vi "GDSLvCLass_ReadClassPropertiesFromFile.vi"(0 "LvClassPathIn":path, 5 "error in (no error)":errorcluster) -> (14 "LvClassPathOut":path, 15 "ClassSettings":T1, 16 "DataFlowClass":bool, 19 "error out":errorcluster)   [LabVIEW 2020]
uses:
  GDSLvCLass_ClassSettingsType.ctl
  GDSLvClass_PlugIn.ctl
  GDSLvClass_PlugInTypes.ctl
  GDSLvClass_ClassTypeSettingNames.ctl
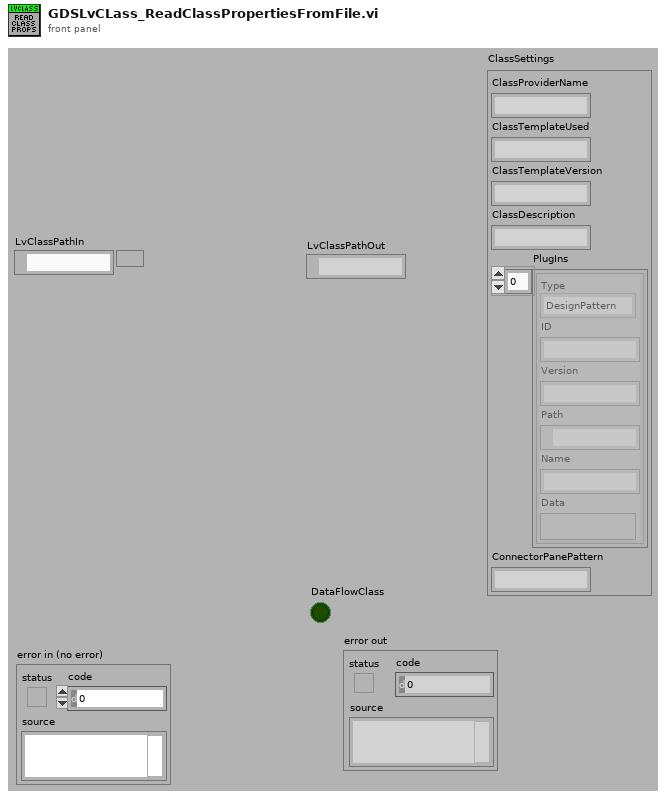
[diagram p1: front panel]
types:
  T1 = typedef "GDSLvCLass_ClassSettingsType.ctl" = cluster{"ClassProviderName":string, "ClassTemplateUsed":string, "ClassTemplateVersion":string, "ClassDescription":string, "PlugIns":T2[], "ConnectorPanePattern":string}
  T2 = typedef "GDSLvClass_PlugIn.ctl" = cluster{"Type":T3, "ID":string, "Version":string, "Path":path, "Name":string, "Data":variant}
  T3 = typedef "GDSLvClass_PlugInTypes.ctl" = enum16{"DesignPattern", "MethodTypes"}
  T4 = typedef "GDSLvClass_ClassTypeSettingNames.ctl" = enum16{"EndevoGOOP_ClassProvider", "EndevoGOOP_TemplateUsed", "EndevoGOOP_TemplateVersion", "EndevoGOOP_PlugIns", "EndevoGOOP_ConnectorPanePattern"}
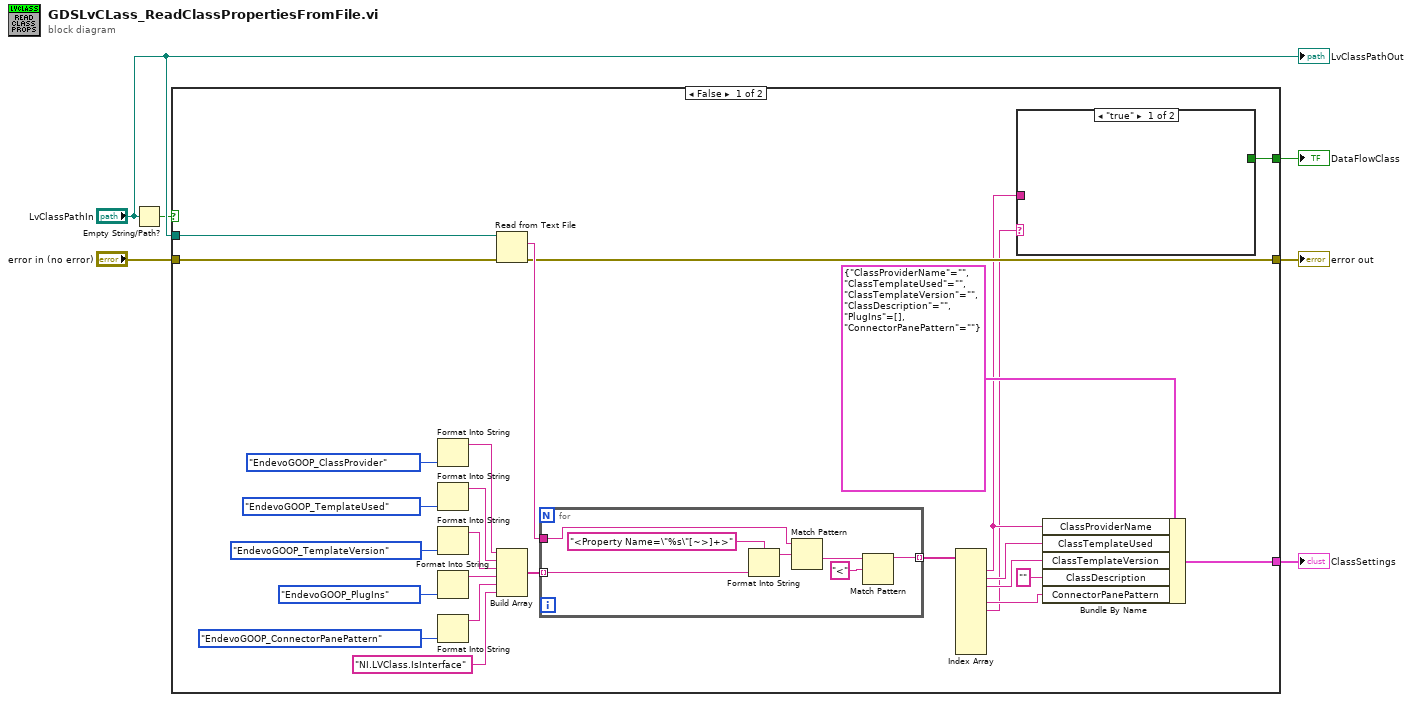
[diagram p0: block diagram]
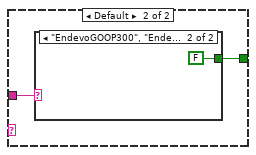
[diagram p2: hidden frame]
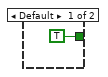
[diagram p3: hidden frame]
diagram:
  n1 = Empty String/Path?(string/path="LvClassPathIn") -> (empty?=w4:bool)
  n2 = case shown="False" w4 {
    tunnel: [w30 w44] -> w6
    tunnel: "LvClassPathIn" -> [w12 _]
    tunnel: "error in (no error)" -> [w18 w44]
    tunnel: [w16 _] -> w2
    tunnel: [w10 _] -> w1
    frame False {
      n3 = Format Into String(GDSLvClass_ClassTypeSettingNames."EndevoGOOP_ClassProvider" ("ClassTypeSettingNames")) -> (resulting string=w28:string)  [unwired: 3 in, 1 out]
      n4 = Format Into String(GDSLvClass_ClassTypeSettingNames."EndevoGOOP_TemplateUsed" ("ClassTypeSettingNames")) -> (resulting string=w26:string)  [unwired: 3 in, 1 out]
      n5 = Format Into String(GDSLvClass_ClassTypeSettingNames."EndevoGOOP_TemplateVersion" ("ClassTypeSettingNames")) -> (resulting string=w24:string)  [unwired: 3 in, 1 out]
      n6 = Format Into String(GDSLvClass_ClassTypeSettingNames."EndevoGOOP_PlugIns" ("ClassTypeSettingNames")) -> (resulting string=w21:string)  [unwired: 3 in, 1 out]
      n7 = Format Into String(GDSLvClass_ClassTypeSettingNames."EndevoGOOP_ConnectorPanePattern" ("ClassTypeSettingNames")) -> (resulting string=w19:string)  [unwired: 3 in, 1 out]
      n8 = Read from Text File(file (use dialog)=w12, error in=w18) -> (text=w32:string, error out=w30:errorcluster)  [unwired: 2 in, 2 out]
      n9 = Build Array(w28, w26, w24, w21, w19, "NI.LVClass.IsInterface" ("element")) -> (w29:string[])
      n10 = for {
        tunnel: w32 -> [w42]
        tunnel: w29 -> [w40] mode=indexing
        tunnel: [w37] -> w31 mode=indexing
        n11 = Format Into String(format string="<Property Name=\"%s\"[~>]+>" ("string"), w40) -> (resulting string=w41:string)  [unwired: 2 in, 1 out]
        n12 = Match Pattern(string=w42, regular expression=w41) -> (after substring=w39:string)  [unwired: 1 in, 3 out]
        n13 = Match Pattern(string=w39, regular expression="<") -> (before substring=w37:string)  [unwired: 1 in, 3 out]
      }
      n14 = Index Array(array=w31) -> (element #1=w11:string, element #2=w15:string, element #3=w14:string, element #5=w8:string, element #6=w7:string)  [unwired: 11 in, 6 out]
      n15 = case shown="\"true\"" w7 {
        tunnel: w11 -> [_ w34]
        tunnel: [_ w33] -> w10
        frame "true" {
        }
        frame Default {
          n16 = case shown="\"EndevoGOOP300\", \"EndevoGOOP400\", \"OpenG100\"" w34 {
            tunnel: [TRUE FALSE] -> w33
            frame Default {
            }
            frame "EndevoGOOP300", "EndevoGOOP400", "OpenG100" {
            }
          }
        }
      }
      n17 = Bundle By Name(cluster=T1 {"ClassProviderName"="", "ClassTemplateUsed"="", "ClassTemplateVersion"="", "ClassDescription"="", "PlugIns"=[], "ConnectorPanePattern"=""} ("ClassSettings"), "ClassProviderName"=w11, "ClassTemplateUsed"=w15, "ClassTemplateVersion"=w14, "ClassDescription"="", "ConnectorPanePattern"=w8) -> (w16:T1)
    }
    frame True {
    }
  }
  "error out" <- w6
  "ClassSettings" <- w2
  "DataFlowClass" <- w1
  "LvClassPathOut" <- "LvClassPathIn"
